vi "Fetch_chirp_waveform_optimized2.vi"(0 "VISA resource name":refnum<visa-resource-name>, 11 "error in (no error)":errorcluster) -> (4 "VISA resource name out":refnum<visa-resource-name>, 6 "Waveform Data":waveform(dbl)(graph), 12 "overall meas time":u32, 15 "error out":errorcluster)   [LabVIEW 2011]
doc: "Returns the waveform that an oscilloscope acquires for a channel you specify. An acquisition that you initiate before calling this VI generates the waveform.\n\nYou first enable channels with the Configure Channel VI. Then you use the Initiate VI to start an acquisition on the enabled channels. An oscilloscope concurrently acquires waveforms for these channels. You must call the Fetch Waveform VI separately to obtain waveforms for each enabled channel. However, you also can call the Read Waveform VI instead of using the above low-level VIs.\n\n<B>Note:</B> Use the Fetch Waveform VI only with other low-level VIs, such as the Initiate VI, the Abort VI, and the Fetch Waveform Measurement VI. High-level VIs such as the Read Waveform VI automatically incorporate the functions of the Initiate VI and the Fetch Waveform VI. The Fetch Waveform VI does not check the status of an instrument."
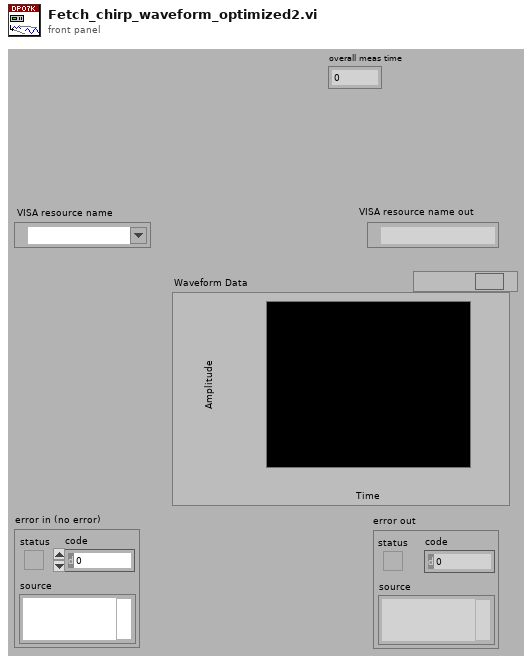
[diagram p1: front panel]
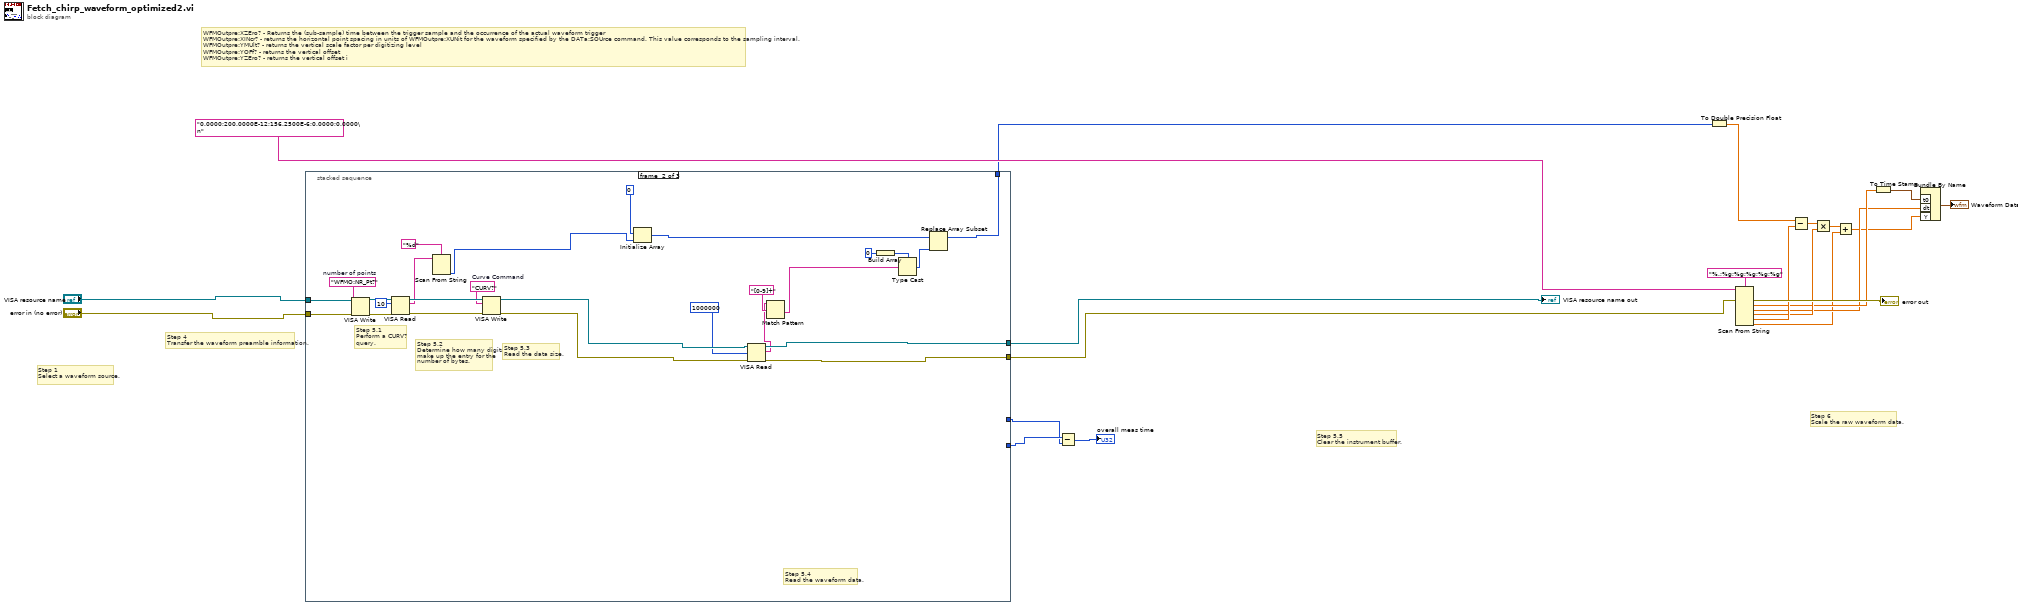
[diagram p0: block diagram]
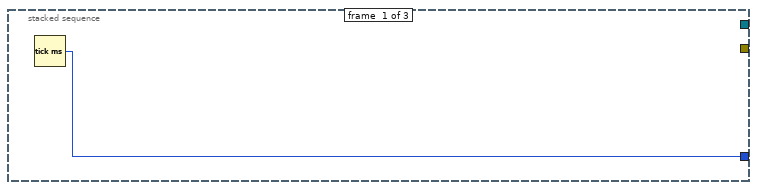
[diagram p2: hidden frame]
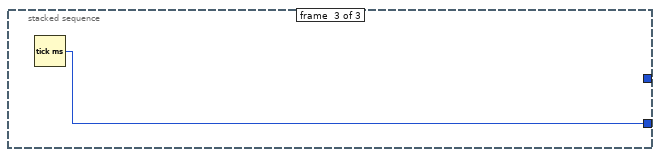
[diagram p3: hidden frame]
diagram:
  # "WFMOutpre:XZEro? - Returns the (sub-sample) time between the trigger sample and the occurrence of the actual waveform trigger\nWFMOutpre:XINcr? - returns the horizontal point spacing in units of WFMOutpre:XUNit for the waveform specified by the DATa:SOUrce command. This value corresponds to the sampling interval.\nWFMOutpre:YMUlt? - returns the vertical scale factor per digitizing level \nWFMOutpre:YOFf? - returns the vertical offset \nWFMOutpre:YZEro? - returns the vertical offset i"
  # "Step 1       \nSelect a waveform source."
  # "Step 6    \nScale the raw waveform data."
  # "Step 5.5    \nClear the instrument buffer."
  # "Step 4\nTransfer the waveform preamble information."
  n1 = stacked-sequence {
    tunnel: [_ w49 _] -> w21
    tunnel: [_ w48 _] -> w20
    tunnel: [_ w44 _] -> w18
    tunnel: "VISA resource name" -> [_ w43 _]
    tunnel: "error in (no error)" -> [_ w42 _]
    tunnel: [w23 _ _] -> w1
    tunnel: [_ _ w50] -> w2
    frame #0 {
      n2 = Tick Count (ms)() -> (millisecond timer value=w23:u32)
    }
    frame #1 {
      w31 = "CURV?"  # Curve Command
      w37 = "WFMO:NR_Pt?"  # number of points
      # "Step 5.4   \nRead the waveform data."
      # "Step 5.3      \nRead the data size."
      # "Step 5.2      \nDetermine how many digits\nmake up the entry for the \nnumber of bytes."
      # "Step 5.1      \nPerform a CURV?\nquery."
      n3 = VISA Write(VISA resource name=w43, write buffer=w37, error in (no error)=w42) -> (VISA resource name out=w38:refnum<visa-resource-name>, error out=w34:errorcluster)  [unwired: 1 out]
      n4 = VISA Read(VISA resource name=w38, byte count=u32 10, error in (no error)=w34) -> (VISA resource name out=w36:refnum<visa-resource-name>, read buffer=w32:string, error out=w35:errorcluster)  [unwired: 1 out]
      n5 = Scan From String(format string="%d", input string=w32) -> (output 1=w46:i32)  [unwired: 3 in, 3 out]
      n6 = VISA Write(VISA resource name=w36, write buffer=w31, error in (no error)=w35) -> (VISA resource name out=w47:refnum<visa-resource-name>, error out=w45:errorcluster)  [unwired: 1 out]
      n7 = Initialize Array(i8 0 ("element"), w46) -> (w40:i8[])
      n8 = VISA Read(VISA resource name=w47, byte count=1000000 ("Buffer Size"), error in (no error)=w45) -> (VISA resource name out=w48:refnum<visa-resource-name>, read buffer=w24:string, error out=w49:errorcluster)  [unwired: 1 out]
      n9 = Match Pattern(string=w24, regular expression="[0-9]+") -> (after substring=w26:string)  [unwired: 1 in, 3 out]
      n10 = Build Array(i8 0) -> (w29:i8[])
      n11 = Type Cast(type=w29, x=w26) -> (*(type *) &x=w27:i8[])
      n12 = Replace Array Subset(array=w40, new element=w27) -> (w44:i8[])  [unwired: 1 in]
    }
    frame #2 {
      n13 = Tick Count (ms)() -> (millisecond timer value=w50:u32)
    }
  }
  "VISA resource name out" <- w20
  n14 = Subtract(x=w2, y=w1) -> (x-y=→"overall meas time":u32)
  n15 = To Double Precision Float(number=w18) -> (double precision float=w19:dbl[])
  n16 = Scan From String(format string="%.;%g;%g;%g;%g;%g", input string="0.0000;200.0000E-12;156.2500E-6;0.0000;0.0000\n" ("read buffer"), error in=w21) -> (error out=→"error out":errorcluster, output 1=w11:dbl, output 2=w9:dbl, output 3=w13:dbl, output 4=w14:dbl, output 5=w7:dbl)  [unwired: 6 in, 2 out]
  n17 = Subtract(x=w19, y=w14) -> (x-y=w15:dbl[])
  n18 = Multiply(x=w15, y=w13) -> (x*y=w8:dbl[])
  n19 = Add(x=w8, y=w7) -> (x+y=w6:dbl[])
  n20 = To Time Stamp(1:w11) -> (0:w10:timestamp)
  n21 = Bundle By Name ("Build Waveform")("t0"=w10, "dt"=w9, "Y"=w6) -> (→"Waveform Data":waveform(dbl))  [unwired: 1 in]
